vi "S2C_Access_Globals.vi"() -> ()   [LabVIEW 2015]
uses:
  <vilib>/addons/database/Connection.llb/Conn ObjectReference.ctl
  S2C_Access_Select.ctl
  <vilib>/addons/database/NI_Database_API.lvlib
panel:
  in  "DB_Ver":string
  out "Changed?":bool
  in  "Info":refnum<vi>
  in  "TblName":refnum<vi>
  in  "Section":refnum<vi>
  in  "TblSelect":refnum<vi>
  in  "VI Ref":refnum<vi>
  in  "TblRef":refnum<vi>
  in  "DSN_File":path=path "C:/Personal/Labview/S2C/Access.dsn"
  out "DB_Ref":T1
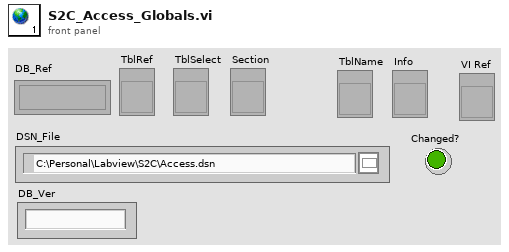
[diagram p1: front panel]
types:
  T1 = typedef "NI_Database_API.lvlib/Conn ObjectReference.ctl" = refnum<k1>
diagram:
